vi "Redis_Create.vi"(0 "reference in":refnum<class "Redis.lvclass">, 5 "Host":string="localhost", 7 "Port":u32=6379, 9 "Authentication":cluster{"Username":string, "Password":string}, 11 "Error In":errorcluster, 12 "UseAuthentication(F)":bool) -> (4 "reference out":refnum<class "Redis.lvclass">, 8 "Connected?":bool, 15 "Error Out":errorcluster)   [LabVIEW 2020, in "Redis.lvclass"]
uses:
  Redis.lvclass
  Redis.lvclass/Redis.ctl
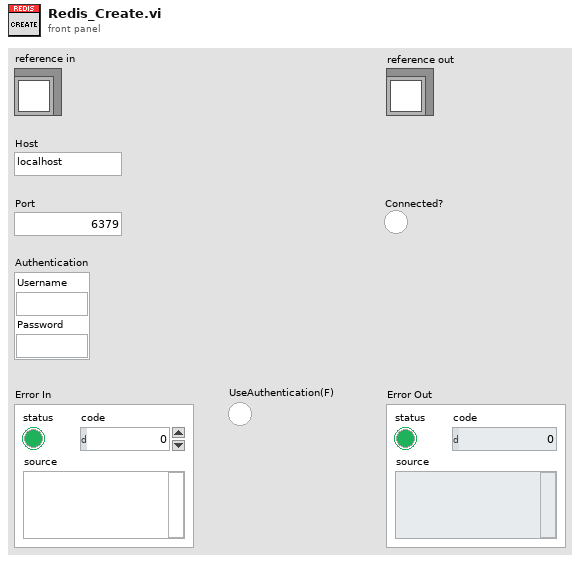
[diagram p1: front panel]
types:
  T1 = typedef "RedisConnection.lvclass/ObjectAttributes.ctl" = cluster{"Port":u32, "Host":string, "Username":string, "Password":string, "UseAuthentication":bool}
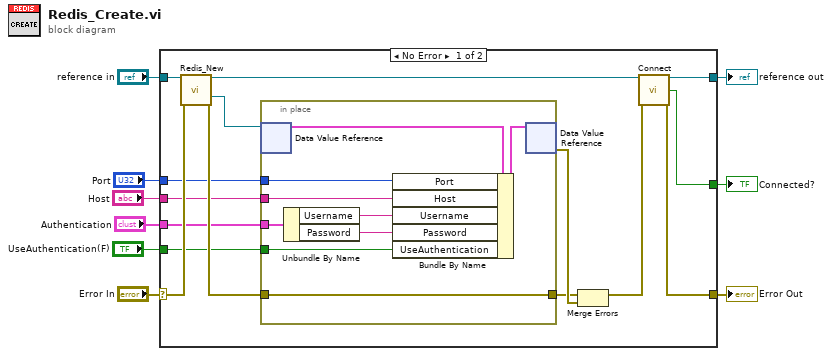
[diagram p0: block diagram]
diagram:
  n1 = case shown="No Error" "Error In" {
    selector: "Error In" -> [w23 w35]
    tunnel: [w11 w35] -> w8
    tunnel: "reference in" -> [w24 w34]
    tunnel: [w13 w34] -> w6
    tunnel: "Port" -> [w18 _]
    tunnel: "Host" -> [w17 _]
    tunnel: "UseAuthentication(F)" -> [w16 _]
    tunnel: "Authentication" -> [w15 _]
    tunnel: [w10 _] -> w1
    frame No Error {
      n2 = call "Redis_New.vi"("reference in"=w24, "Error In"=w23) -> ("reference out"=w14:refnum<class "Redis.lvclass">, "DVRRefOut"=w21:refnum<data-value>, "Error Out"=w20:errorcluster)  [unwired: 10 in, 1 out]
      n3 = in-place {
        in-place-border: w20 -> [w31]
        in-place-border: [w31] -> w19
        in-place-border: w18 -> [w30]
        in-place-border: w17 -> [w29]
        in-place-border: w16 -> [w28]
        in-place-border: w15 -> [w27]
        n4 = in-place-dvr #1(w21) -> (w32:T1)  [unwired: 1 out]
        n5 = Unbundle By Name(w27) -> ("Username"=w26:string, "Password"=w25:string)
        n6 = Bundle By Name(cluster=w32, "Port"=w30, "Host"=w29, "Username"=w26, "Password"=w25, "UseAuthentication"=w28) -> (w33:T1)
        n7 = in-place-dvr #1(w33) -> (w22:errorcluster)  [unwired: 1 out]
      }
      n8 = Merge Errors(w19, w22) -> (w12:errorcluster)
      n9 = call "Connect.vi"("reference in"=w14, "Error In"=w12) -> ("reference out"=w13:refnum<class "Redis.lvclass">, "Connected?"=w10:bool, "Error Out"=w11:errorcluster)  [unwired: 11 in]
    }
    frame Error {
      # "VI-TechBaseTemplate_Simple_4x4x4"
    }
  }
  "Error Out" <- w8
  "reference out" <- w6
  "Connected?" <- w1
